vi "UART Receive Data.vi"(0 "UART Driver in":refnum<class "UART Driver.lvclass">, 1 "Channel Number":u8=1, 5 "Rx byte count":u32, 9 "timeout (s)":dbl=10.0, 11 "error in":errorcluster) -> (4 "UART Driver out":refnum<class "UART Driver.lvclass">, 6 "Receive Data":string, 15 "error out":errorcluster)   [LabVIEW 2012, in "UART_Host_Driver.lvlib" / "UART Driver.lvclass"]
uses:
  UART Driver.lvclass
  Typedefs/FPGA VI Reference.ctl
  UART Driver.lvclass/UART Driver.ctl
  <vilib>/Utility/error.llb/Error Cluster From Error Code.vi
  <vilib>/rvi/errors/niLvFpgaAdjustHostInterfaceError.vi
  <vilib>/rvi/interface/nirviMethod/nirviMethod.xnode
  <vilib>/ErrorRing/Error Ring.xnode
  UART_Host_Driver.lvlib
  <vilib>/FPGAPlugInAG/Dynamic/niLvFpga_ReadFifo_Dynamic.vi
  <vilib>/rvi/errors/niLvFpgaMergeErrorWithErrorCode.vi
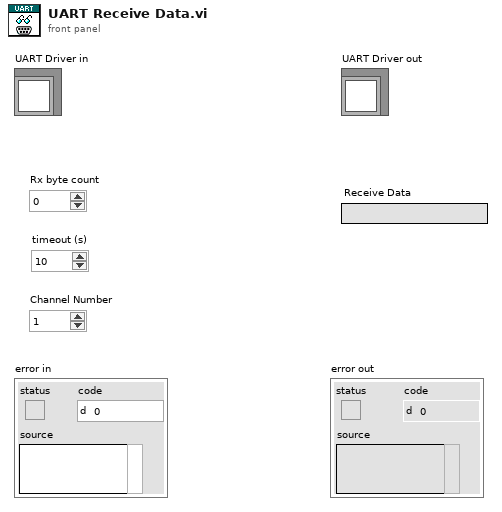
[diagram p1: front panel]
types:
  T1 = typedef "UART_Host_Driver.lvlib/FPGA VI Reference.ctl" = refnum<k20>
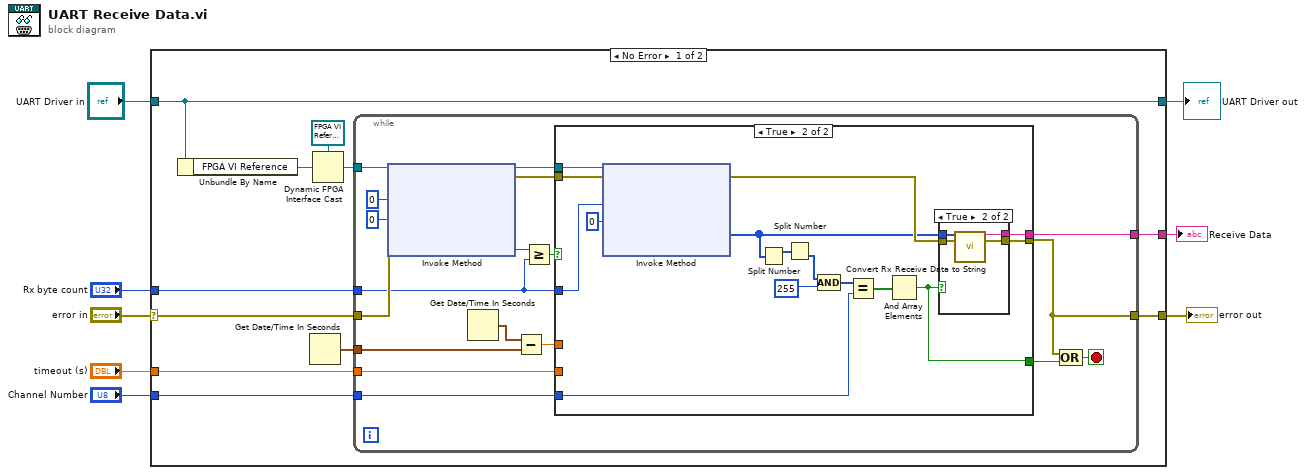
[diagram p0: block diagram]
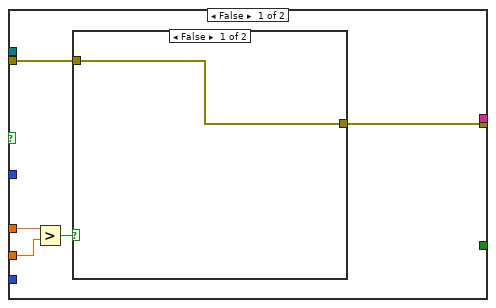
[diagram p2: hidden frame]
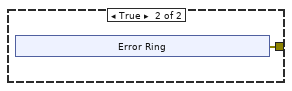
[diagram p3: hidden frame]
diagram:
  n1 = case shown="No Error" "error in" {
    selector: "error in" -> [w15 w71]
    tunnel: [w14 w71] -> w7
    tunnel: [w19 w70] -> w5
    tunnel: "UART Driver in" -> [w19 w70]
    tunnel: "Rx byte count" -> [w9 _]
    tunnel: [w13 _] -> w4
    tunnel: "timeout (s)" -> [w12 _]
    tunnel: "Channel Number" -> [w10 _]
    frame No Error {
      n2 = Unbundle By Name(w19) -> ("FPGA VI Reference"=w18:refnum<k20>)
      n3 = Get Date/Time In Seconds() -> (seconds since 1Jan1904=w11:timestamp)
      n4 = Dynamic FPGA Interface Cast(Session In=T1 refnum ("FPGA VI Reference"), Type=w18) -> (Session Out=w16:T1)
      n5 = while {
        tunnel: w16 -> [w37]
        tunnel: w15 -> [w36]
        tunnel: w9 -> [w30]
        tunnel: [w20] -> w14
        tunnel: [w21] -> w13
        tunnel: w12 -> [w24]
        tunnel: w11 -> [w27]
        tunnel: w10 -> [w22]
        stop <- w23 stop-if-true
        n6 = xnode "Invoke Method"("FPGA VI Reference In"=w37, "error in"=w36, "Number of Elements"=u32 0, "Timeout (ms)"=0) -> ("FPGA VI Reference Out"=w33:T1, "error out"=w29:errorcluster, "Elements Remaining"=w32:u32)  [unwired: 1 out]
        n7 = Get Date/Time In Seconds() -> (seconds since 1Jan1904=w26:timestamp)
        n8 = Subtract(x=w26, y=w27) -> (x-y=w25:dbl)
        n9 = Greater Or Equal?(x=w32, y=w30) -> (x >= y?=w31:bool)
        n10 = case shown="True" w31 {
          tunnel: w33 -> [_ w64]
          tunnel: w30 -> [_ w63]
          tunnel: w29 -> [w39 w61]
          tunnel: [w38 w52] -> w20
          tunnel: [_ w50] -> w28
          tunnel: w25 -> [w42 _]
          tunnel: w24 -> [w41 _]
          tunnel: w22 -> [_ w56]
          tunnel: [_ w53] -> w21
          frame False {
            n11 = Greater?(x=w42, y=w41) -> (0:w40:bool)
            n12 = case shown="False" w40 {
              tunnel: w39 -> [w43 _]
              tunnel: [w43 w44] -> w38
              frame False {
              }
              frame True {
                n13 = xnode "Error Ring"() -> ("error out"=w44:errorcluster)
              }
            }
          }
          frame True {
            n14 = xnode "Invoke Method"("FPGA VI Reference In"=w64, "error in"=w61, "Number of Elements"=w63, "Timeout (ms)"=0) -> ("error out"=w55:errorcluster, "Data"=w54:u32[])  [unwired: 2 out]
            n15 = Split Number(x=w54) -> (hi(x)=w58:u16[])  [unwired: 1 out]
            n16 = Split Number(x=w58) -> (lo(x)=w57:u8[])  [unwired: 1 out]
            n17 = Compound Arithmetic op=AND(w57, u8 255 ("Numeric")) -> (w59:u8[])
            n18 = Equal?(x=w59, y=w56) -> (x = y?=w51:bool[])
            n19 = And Array Elements(Boolean array=w51) -> (logical AND=w50:bool)
            n20 = case shown="True" w50 {
              tunnel: w55 -> [w65 w69]
              tunnel: w54 -> [_ w68]
              tunnel: [_ w67] -> w53
              tunnel: [w65 w66] -> w52
              frame False {
              }
              frame True {
                n21 = call "Convert Rx Receive Data to String.vi"("RX_data"=w68, "error in"=w69) -> ("String"=w67:string, "error out"=w66:errorcluster)  [unwired: 12 in]
              }
            }
          }
        }
        n22 = Compound Arithmetic op=OR(w20, w28) -> (w23:bool)
      }
    }
    frame Error {
    }
  }
  "error out" <- w7
  "UART Driver out" <- w5
  "Receive Data" <- w4
